vi "p1.vi"() -> ()   [LabVIEW 2021, in "d15.lvlib"]
uses:
  d15.lvlib
  AOC/AOC.lvlib
panel:
  in  "Example":string="Sensor at x=2, y=18: closest beacon is at x=-2, y=15\nSensor at x=9, y=16: closest beacon is at x=10, y=16\nSensor at x=13, y=2: closest beacon is at x=15, y=3\nSensor at x=12, y=14: closest beacon is at x=10, y=16\nSensor at x=10, y=20: closest beacon is at x=10, y=16\nSensor at x=14, y=17: closest beacon is at x=10, y=16\nSensor at x=8, y=7: closest beacon is at x=2, y=10\nSensor at x=2, y=0: closest beacon is at x=2, y=10\nSensor at x=0, y=11: closest beacon is at x=2, y=10\nSensor at x=20, y=14: closest beacon is at x=25, y=17\nSensor at x=17, y=20: closest beacon is at x=21, y=22\nSensor at x=16, y=7: closest beacon is at x=15, y=3\nSensor at x=14, y=3: closest beacon is at x=15, y=3\nSensor at x=20, y=1: closest beacon is at x=15, y=3"
  in  "Example":bool
  out "Answer":i64=4737443
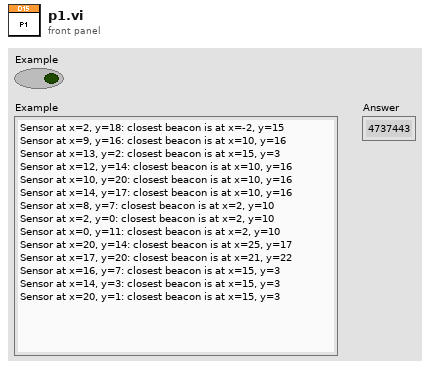
[diagram p1: front panel]
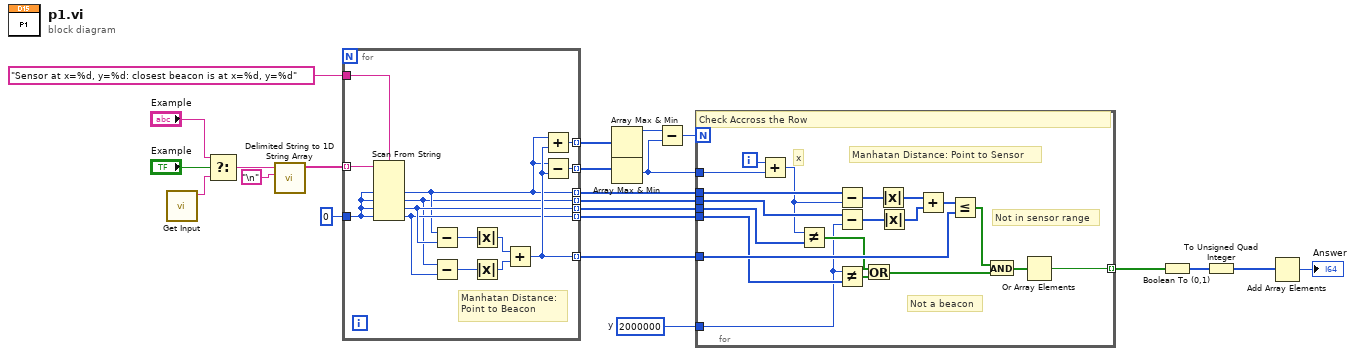
[diagram p0: block diagram]
diagram:
  w4 = i64 2000000  # y
  n1 = call "Get Input.vi"() -> ("Input"=w23:string)  [unwired: 11 in]
  n2 = Select(t="Example", s="Example", f=w23) -> (s? t:f=w22:string)
  n3 = call <vilib>:"Delimited String to 1D String Array.vi"("delimiter"="\n", "delimited string"=w22) -> ("string array"=w18:string[])  [unwired: 9 in]
  n4 = for {
    tunnel: w18 -> [w37] mode=indexing
    tunnel: "Sensor at x=%d, y=%d: closest beacon is at x=%d, y=%d" ("format string") -> [w36]
    tunnel: i64 0 ("default value 1") -> [w35]
    tunnel: [w25] -> w8 mode=indexing
    tunnel: [w32] -> w15 mode=indexing
    tunnel: [w31] -> w14 mode=indexing
    tunnel: [w24] -> w11 mode=indexing
    tunnel: [w30] -> w12 mode=indexing
    tunnel: [w29] -> w6 mode=indexing
    tunnel: [w28] -> w7 mode=indexing
    # "Manhatan Distance:\nPoint to Beacon"
    n5 = Scan From String(format string=w36, input string=w37, default 1=w35, default 2=w35, default 3=w35, default 4=w35) -> (output 1=w25:i64, output 2=w24:i64, output 3=w29:i64, output 4=w28:i64)  [unwired: 2 in, 3 out]
    n6 = Subtract(x=w25, y=w29) -> (x-y=w34:i64)
    n7 = Subtract(x=w24, y=w28) -> (x-y=w33:i64)
    n8 = Absolute Value(x=w34) -> (abs(x)=w27:i64)
    n9 = Absolute Value(x=w33) -> (abs(x)=w26:i64)
    n10 = Add(x=w27, y=w26) -> (x+y=w30:i64)
    n11 = Add(x=w25, y=w30) -> (x+y=w32:i64)
    n12 = Subtract(x=w25, y=w30) -> (x-y=w31:i64)
  }
  n13 = Array Max & Min(array=w15) -> (max value=w13:i64)  [unwired: 3 out]
  n14 = Array Max & Min(array=w14) -> (min value=w5:i64)  [unwired: 3 out]
  n15 = Subtract(x=w13, y=w5) -> (x-y=w9:i64)
  n16 = for {
    N: w9 -> [_]
    tunnel: w12 -> [w56]
    tunnel: w11 -> [w55]
    tunnel: w8 -> [w57]
    tunnel: w7 -> [w53]
    tunnel: w6 -> [w52]
    tunnel: w5 -> [w50]
    tunnel: w4 -> [w39]
    tunnel: [w38] -> w2 mode=indexing
    i -> [w54]
    # "Not a beacon"
    # "Not in sensor range"
    # "Manhatan Distance: Point to Sensor"
    # "x"
    # "Check Accross the Row"
    n17 = Add(x=w54, y=w50) -> (x+y=w51:i64)
    n18 = Not Equal?(x=w51, y=w52) -> (x != y?=w45:bool[])
    n19 = Subtract(x=w57, y=w51) -> (x-y=w49:i64[])
    n20 = Subtract(x=w55, y=w39) -> (x-y=w48:i64[])
    n21 = Not Equal?(x=w39, y=w53) -> (x != y?=w41:bool[])
    n22 = Or(x=w45, y=w41) -> (x .or. y?=w40:bool[])
    n23 = Absolute Value(x=w49) -> (abs(x)=w43:i64[])
    n24 = Absolute Value(x=w48) -> (abs(x)=w44:i64[])
    n25 = Add(x=w43, y=w44) -> (x+y=w47:i64[])
    n26 = Less Or Equal?(x=w47, y=w56) -> (x <= y?=w46:bool[])
    n27 = And(x=w46, y=w40) -> (x .and. y?=w42:bool[])
    n28 = Or Array Elements(Boolean array=w42) -> (logical OR=w38:bool)
  }
  n29 = Boolean To (0,1)(Boolean=w2) -> (0, 1=w3:i16[])
  n30 = To Unsigned Quad Integer(1:w3) -> (0:w1:u64[])
  n31 = Add Array Elements(numeric array=w1) -> (sum=→"Answer":u64)
